vi "SizeSpecification.vi"(10 "Size":T1) -> (3 "SizeSpecification":refnum<class "SizeSpecification.lvclass">)   [LabVIEW 2018, in "SizeSpecification.lvclass"]
uses:
  SizeSpecification.lvclass
  Product/Size.ctl
  SizeSpecification.lvclass/SizeSpecification.ctl
  Product/Product.lvclass
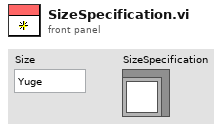
[diagram p1: front panel]
types:
  T1 = typedef "Product.lvclass/Size.ctl" = enum16{"Yuge", "Big", "Medium", "Small"}
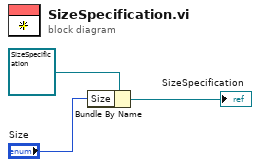
[diagram p0: block diagram]
diagram:
  n1 = Bundle By Name(cluster=refnum<class "SizeSpecification.lvclass"> refnum ("SizeSpecification.lvclass"), "Size"="Size") -> (→"SizeSpecification":refnum<class "SizeSpecification.lvclass">)
